vi "lv_opencv_demo.vi"() -> ()   [LabVIEW 2021]
uses:
  lv_ov_dll.dll
panel:
  out "detection":T1(plugin-control)
  out "detections":sgl[](array[numeric])
  out "Original":T1(plugin-control)
  out "error out":errorcluster
  # "[class_id, score, x1, y1, x2, y2]"
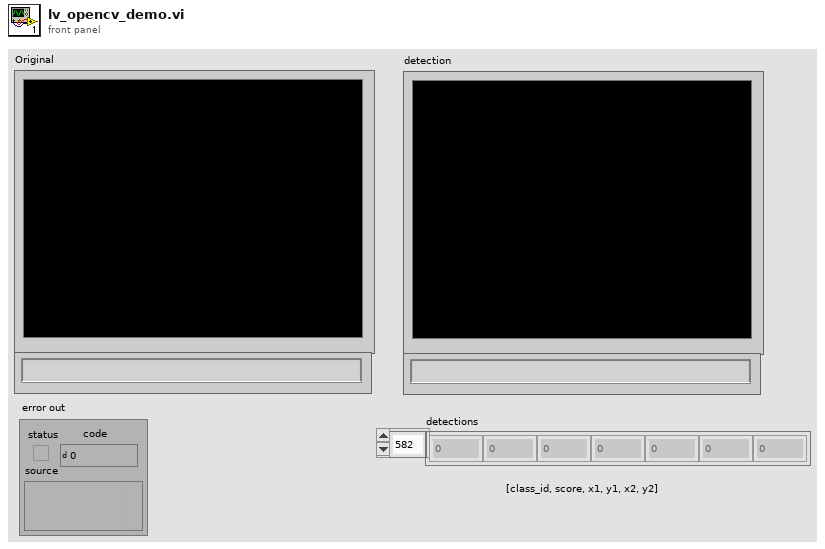
[diagram p1: front panel]
types:
  T1 = typedef "IMAQ Image.ctl" = refnum<image>
  T2 = typedef "Image Type" = u32
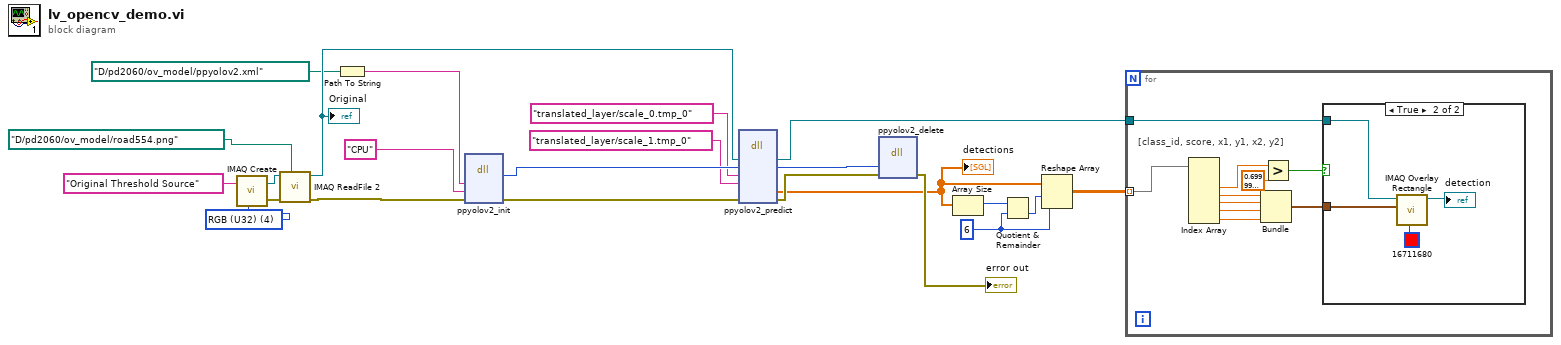
[diagram p0: block diagram]
diagram:
  w5 = 6 ("dimension size")
  w19 = T2 4 items=["Grayscale (U8)", "Grayscale (I16)", "Grayscale (SGL)", "Complex (CSG)", "RGB (U32)", "HSL (U32)", "RGB (U64)", "Grayscale (U16)"] ("Image Type")
  n1 = call "IMAQ Create"("Image Name"="Original Threshold Source", "Image Type"=w19) -> ("New Image"=w22:T1, "error out"=w21:errorcluster)  [unwired: 3 in]
  n2 = call "IMAQ ReadFile 2"("File Path"=path "D:/pd2060/ov_model/road554.png" ("path"), "error in (no error)"=w21, "Image"=w22) -> ("error out"=w3:errorcluster, "Image Out"=w20:T1)  [unwired: 4 in, 3 out]
  "Original" <- w20
  n3 = Path To String(path=path "D:/pd2060/ov_model/ppyolov2.xml") -> (string=w17:string)
  n4 = dll-call lib="D:/pd2060/lv_ov_wrapper/lv_ov_dll/bin/x64/Release/lv_ov_dll.dll" fn="ppyolov2_init"("model_xml_file"=w17, "device_name"="CPU", "err"=w3) -> ("return type"=w14:u64, "err"=w15:errorcluster)  [unwired: 5 in, 2 out]
  n5 = dll-call lib="D:/pd2060/lv_ov_wrapper/lv_ov_dll/bin/x64/Release/lv_ov_dll.dll" fn="ppyolov2_predict"("sourceHandle"=w20, "pInferEngine"=w14, "bbox_name"="translated_layer/scale_0.tmp_0", "bbox_num_name"="translated_layer/scale_1.tmp_0", "err"=w15) -> ("sourceHandle"=w2:T1, "pInferEngine"=w12:u64, "detections"=w8:sgl[], "err"=w10:errorcluster)  [unwired: 7 in, 2 out]
  "detections" <- w8
  n6 = dll-call lib="D:/pd2060/lv_ov_wrapper/lv_ov_dll/bin/x64/Release/lv_ov_dll.dll" fn="ppyolov2_delete"("pInferEngine"=w12, "err"=w10) -> ("err"=→"error out":errorcluster)  [unwired: 5 in, 2 out]
  n7 = Array Size(array=w8) -> (size(s)=w7:i32)
  n8 = Quotient & Remainder(x=w7, y=w5) -> (floor(x/y)=w6:i32)  [unwired: 1 out]
  n9 = Reshape Array(w8, w6, w5) -> (w4:sgl[][])
  n10 = for {
    tunnel: w4 -> [w33] mode=indexing
    tunnel: w2 -> [w24]
    # "[class_id, score, x1, y1, x2, y2]"
    n11 = Index Array(array=w33) -> (element #2=w32:sgl, element #3=w29:sgl, element #4=w28:sgl, element #5=w27:sgl, element #6=w26:sgl)  [unwired: 6 in, 1 out]
    n12 = Bundle(w29, w28, w27, w26) -> (w25:cluster{sgl, sgl, sgl, sgl})  [unwired: 1 in]
    n13 = Greater?(x=w32, y=sgl 0.7) -> (0:w30:bool)
    n14 = case shown="True" w30 {
      tunnel: w25 -> [_ w36]
      tunnel: w24 -> [_ w35]
      frame False {
      }
      frame True {
        n15 = call "IMAQ Overlay Rectangle"("Color"=u32 16711680, "Rectangle"=w36, "Image"=w35) -> ("Image Out"=→"detection":T1)  [unwired: 7 in, 1 out]
      }
    }
  }
